vi "(SubVI)I2C_8Bit-8Bit_Write_Single.vi"(5 "Log Ref":refnum<vi>, 7 "Clock":T1=enum."400kHz", 8 "error in (no error)":errorcluster caption="에러 입력(에러 없음)", 9 "Data to Write":u8, 10 "Address":u8, 11 "ID":u8) -> (0 "error out":errorcluster caption="에러 출력", 2 "Log":string)   [LabVIEW 2020]
uses:
  Controls/(Ctrl)I2C_Clock.ctl
  Serial/Controls/(Ctrl)Serial_Write Read Option.ctl
  Controls/(Ctrl)I2C_RW.ctl
  Controls/(Ctrl)I2C_Data Size.ctl
  Variables/(Var)System Variables.vi
  Serial/Instance VIs/(SubVI)Serial_Write-Read.vi
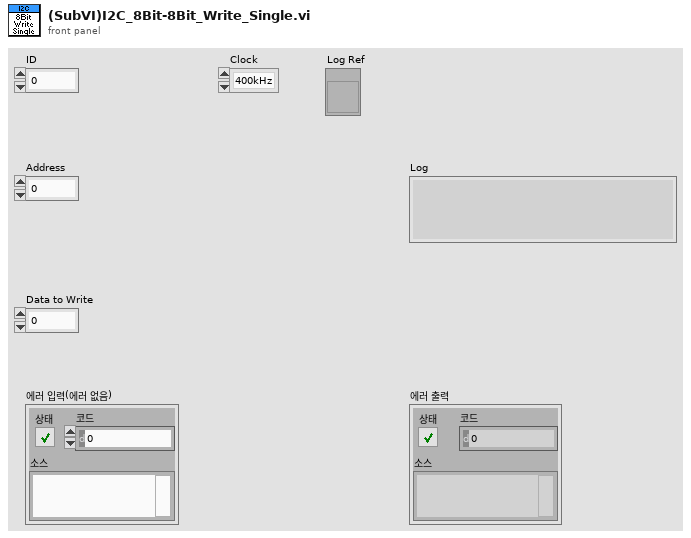
[diagram p1: front panel]
types:
  T1 = typedef "(Ctrl)I2C_Clock.ctl" = enum8{"1MHz", "2MHz", "3MHz", "400kHz"}
  T2 = typedef "(Ctrl)I2C_Data Size.ctl" = enum16{"8Bit_8Bit", "16Bit_16Bit", "16Bit_8Bit"}
  T3 = typedef "(Ctrl)I2C_RW.ctl" = enum16{"Read", "Write"}
  T4 = typedef "(Ctrl)Serial_Write Read Option.ctl" = cluster{"Echo Request":bool, "Header Verification":bool, "Checksum Verification":bool, "User Code Verifiaction":bool}
  T5 = typedef "IC I2C Clock Rate.ctl" = enum8{"50khz", "100khz", "400khz", "1Mhz", "1.2Mhz"}
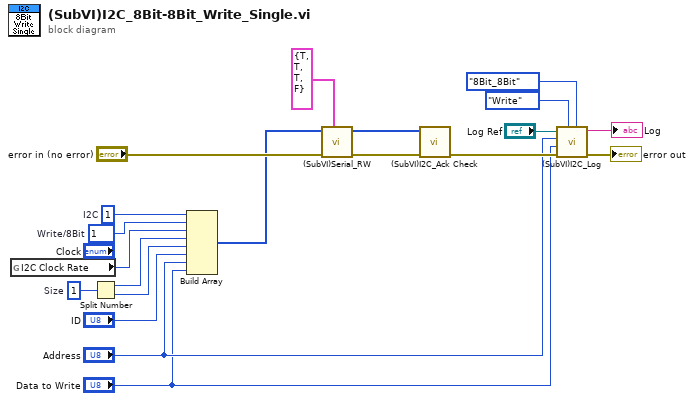
[diagram p0: block diagram]
diagram:
  w13 = u16 1  # Size
  w18 = u8 1  # Write/8Bit
  w19 = u8 1  # I2C
  n1 = global read "(Var)System Variables.vi" "I2C Clock Rate"() -> (w1:T5)
  n2 = Split Number(x=w13) -> (hi(x)=w17:u8, lo(x)=w16:u8)
  n3 = Build Array(w19, w18, w1, w17, w16, "ID", "Address", "Data to Write") -> (w2:u8[])
  n4 = call-poly "(SubVI)Serial_RW.vi"("Option"=T4 {"Echo Request"=TRUE, "Header Verification"=TRUE, "Checksum Verification"=TRUE, "User Code Verifiaction"=FALSE}, "error in (no error)"="error in (no error)", "Data to Write"=w2) -> ("error out"=w10:errorcluster, "Read Data"=w11:u8[])  [unwired: 6 in, 1 out]
  n5 = call "(SubVI)I2C_Ack Check.vi"("에러 입력(에러 없음)"=w10, "Read Data"=w11) -> ("에러 출력"=w14:errorcluster)  [unwired: 8 in, 1 out]
  n6 = call "(SubVI)I2C_Log.vi"("Data Size"=(Ctrl)I2C_Data_Size."8Bit_8Bit", "R/W"=(Ctrl)I2C_RW."Write", "error in (no error)"=w14, "Data"="Data to Write", "Address"="Address", "Log Ref"="Log Ref") -> ("error out"=→"error out":errorcluster, "Log"=→"Log":string)  [unwired: 4 in]
